vi "Front Panel2A.vi"() -> ()   [LabVIEW 2021]
uses:
  GL_TempDspl.vi
  GL_SetpointDispl.vi
  GL_SamplerateDispl.vi
  GL_HeaterOn.vi
  GL_heaterdisplay.vi
  GL_MHeaterDisplay.vi
  GL_Pgain.vi
  GL_Ireset.vi
  GL_Drate.vi
  GL_TempUnits.vi
panel:
  in  "SETUP / ADJUST":bool
  out "TEMPERATURE\nDisplay":dbl format="%.3f"
  out "unit":enum16{"K", "Ohms", "C", "F"}(ring)
  in  "STOP":bool=TRUE
  out "SET POINT":dbl min=0.0 max=450.0 step=0.0001 format="%.4f"
  out "SAMPLE RATE":dbl=0.292 min=0.0 max=600.0 step=0.0001 format="%.4f"
  out "Array":bool[](array[boolean])
  out "HEATER ON":bool
  out "MANUAL HEATER DISPLAY":dbl(slide) caption="AMP" min=0.0 max=5.0 scale=0.0..5.0
  out "P":dbl min=0.0 max=450.0 step=0.0001 format="%.4f"
  out "I":dbl min=0.0 max=450.0 step=0.0001 format="%.4f"
  out "D":dbl min=0.0 max=450.0 step=0.0001 format="%.4f"
  # "e"
  # "e"
  # "TEMPERATURE \nREMOTE TEMPERATURE CONTROLLER"
  # "TEMPERATURE \nREMOTE TEMPERATURE CONTROLLER"
  # "SET  POINT"
  # "SET  POINT"
  # "SAMPLE RATE"
  # "remote heater control\nnot functioning"
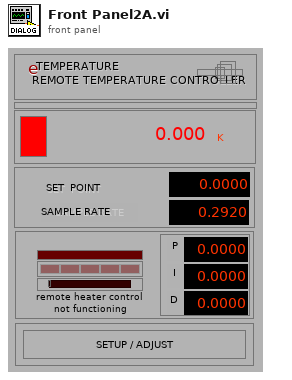
[diagram p1: front panel]
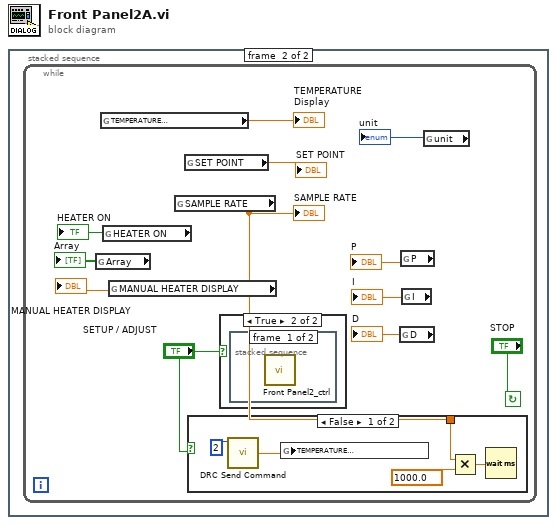
[diagram p0: block diagram]
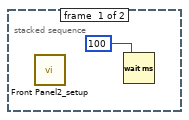
[diagram p2: hidden frame]
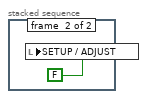
[diagram p5: hidden frame]
diagram:
  n1 = stacked-sequence {
    frame #0 {
      n2 = call "Front Panel2_setup.vi"() -> ()  [unwired: 3 in, 1 out]
      n3 = Wait (ms)(milliseconds to wait=100) -> ()  [unwired: 1 out]
    }
    frame #1 {
      n4 = while {
        stop <- "STOP" continue-if-true
        n5 = global read "GL_heaterdisplay.vi" "Array"() -> (→"Array":bool[])
        n6 = global read "GL_TempDspl.vi" "TEMPERATURE\nDisplay"() -> (→"TEMPERATURE\nDisplay":dbl)
        n7 = global read "GL_HeaterOn.vi" "HEATER ON"() -> (→"HEATER ON":bool)
        n8 = global read "GL_MHeaterDisplay.vi" "MANUAL HEATER DISPLAY"() -> (→"MANUAL HEATER DISPLAY":dbl)
        n9 = global read "GL_SamplerateDispl.vi" "SAMPLE RATE"() -> (w3:dbl)
        "SAMPLE RATE" <- w3
        n10 = global read "GL_SetpointDispl.vi" "SET POINT"() -> (→"SET POINT":dbl)
        n11 = case shown="False" "SETUP / ADJUST" {
          tunnel: w3 -> [w14 _]
          frame False {
            n12 = call "DRC Send Command.vi"("Command"=2) -> ("Output"=w18:dbl)  [unwired: 3 in, 2 out]
            n13 = global write "GL_TempDspl.vi" "TEMPERATURE\nDisplay"(w18) -> ()
            n14 = Multiply(x=w14, y=1000.0) -> (x*y=w15:dbl)
            n15 = Wait (ms)(milliseconds to wait=w15) -> ()  [unwired: 1 out]
          }
          frame True {
          }
        }
        n16 = case shown="True" "SETUP / ADJUST" {
          frame False {
          }
          frame True {
            n17 = stacked-sequence {
              frame #0 {
                n18 = call "Front Panel2_ctrl.vi"() -> ()  [unwired: 2 in, 1 out]
              }
              frame #1 {
                n19 = local write "SETUP / ADJUST"(FALSE) -> ()
              }
            }
          }
        }
        n20 = global read "GL_Drate.vi" "D"() -> (→"D":dbl)
        n21 = global read "GL_Pgain.vi" "P"() -> (→"P":dbl)
        n22 = global read "GL_Ireset.vi" "I"() -> (→"I":dbl)
        n23 = global read "GL_TempUnits.vi" "unit"() -> (→"unit":enum16{"K", "Ohms", "C", "F"})
      }
    }
  }
